vi "Juicer-Init.vi"(7 "Device reference":refnum<vi>, 8 "error in (no error)":errorcluster, 10 "OutputRequest event ref":T1, 11 "InputData reference":refnum<vi>) -> (0 "error out":errorcluster, 2 "OutputRequest (dup)":T1, 3 "InputData (dup)":refnum<vi>)   [LabVIEW 2015]
doc: "Initializes a juicer object. Wire its reference to the \"Device reference\" input.\n\nInputData reference: create reference from Main VI\nOutputRequest event ref: get this from Rack-Init\n\nThe outputs are just duplicates to make it easier to call a bunch of Device-Init functions."
uses:
  Typedefs/Juicer.ctl
  Rack/Typedefs/OutputRequest refnum.ctl
  Rack/Typedefs/OutputRequest.ctl
  Rack/Typedefs/InputData cluster.ctl
  Rack/Methods/Port drivers/DigitalInput-DataCluster.ctl
panel:
  # "(must be on same NI card)"
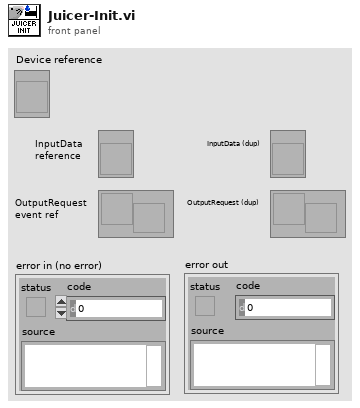
[diagram p1: front panel]
types:
  T1 = typedef "OutputRequest refnum.ctl" = refnum<user-event>
  T2 = typedef "Juicer.ctl" = cluster{"Mode":enum16{"Off", "Juice/reward", "Water flush", "Air purge"}, "Settings":cluster{"Bleed #1 port index":i32, "Bleed #1 port name":string, "Bleed #2 port name":string, "Bleed #2 port index":i32, "Flush port name":string, "Flush port index":i32, "Purge port name":string, "Purge port index":i32, "Timestamp port name":string}, "OutputRequest event ref":T1, "InputData reference":refnum<vi>}
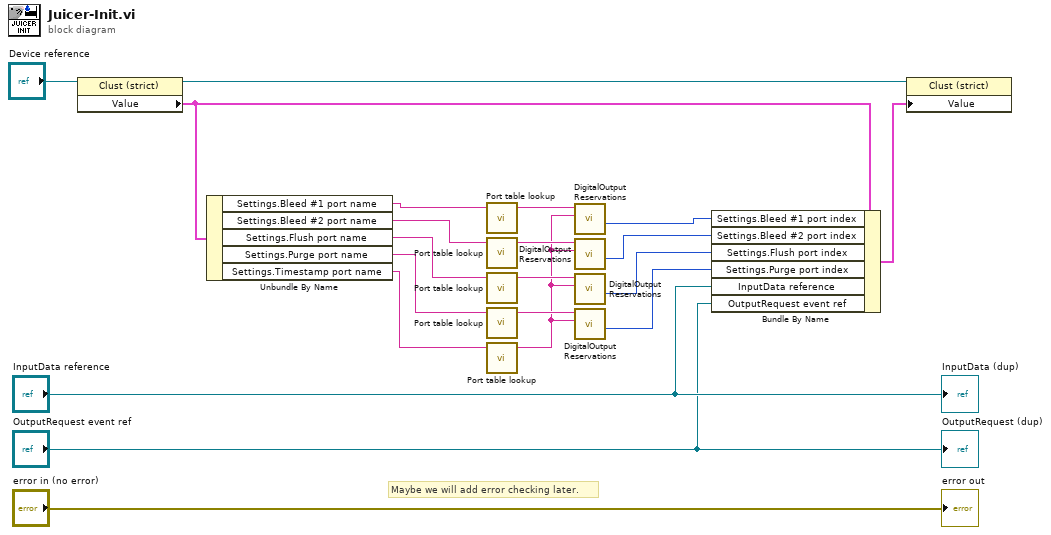
[diagram p0: block diagram]
diagram:
  # "Maybe we will add error checking later."
  n1 = property class="Clust (strict)"(reference="Device reference") -> (reference out=w5:refnum<vi>, "Value"=w10:T2)  [unwired: 1 in, 1 out]
  n2 = Unbundle By Name(w10) -> ("Settings.Bleed #1 port name"=w12:string, "Settings.Bleed #2 port name"=w13:string, "Settings.Flush port name"=w14:string, "Settings.Purge port name"=w15:string, "Settings.Timestamp port name"=w16:string)
  n3 = call "Port table lookup.vi"("Port name"=w12) -> ("Line"=w18:tag)  [unwired: 3 in, 1 out]
  n4 = call "Port table lookup.vi"("Port name"=w13) -> ("Line"=w17:tag)  [unwired: 3 in, 1 out]
  n5 = call "Port table lookup.vi"("Port name"=w14) -> ("Line"=w20:tag)  [unwired: 3 in, 1 out]
  n6 = call "Port table lookup.vi"("Port name"=w15) -> ("Line"=w19:tag)  [unwired: 3 in, 1 out]
  n7 = call "Port table lookup.vi"("Port name"=w16) -> ("Line"=w11:tag)  [unwired: 3 in, 1 out]
  n8 = call "DigitalOutput Reservations.vi"("Timestamp line"=w11, "Line"=w18) -> ("Index assigned"=w9:i32)  [unwired: 2 in, 3 out]
  n9 = call "DigitalOutput Reservations.vi"("Timestamp line"=w11, "Line"=w17) -> ("Index assigned"=w8:i32)  [unwired: 2 in, 3 out]
  n10 = call "DigitalOutput Reservations.vi"("Timestamp line"=w11, "Line"=w20) -> ("Index assigned"=w7:i32)  [unwired: 2 in, 3 out]
  n11 = call "DigitalOutput Reservations.vi"("Timestamp line"=w11, "Line"=w19) -> ("Index assigned"=w6:i32)  [unwired: 2 in, 3 out]
  n12 = Bundle By Name(cluster=w10, "Settings.Bleed #1 port index"=w9, "Settings.Bleed #2 port index"=w8, "Settings.Flush port index"=w7, "Settings.Purge port index"=w6, "InputData reference"="InputData reference", "OutputRequest event ref"="OutputRequest event ref") -> (w4:T2)
  n13 = property class="Clust (strict)"(reference=w5, "Value"=w4) -> ()  [unwired: 1 in, 2 out]
  "error out" <- "error in (no error)"
  "OutputRequest (dup)" <- "OutputRequest event ref"
  "InputData (dup)" <- "InputData reference"
